vi "Destroy.vi"(8 "error in (no error)":errorcluster, 11 "reference in":refnum<class "GOOP4_Sub.lvclass">) -> (0 "error out":errorcluster, 3 "reference out":refnum<class "GOOP4_Sub.lvclass">)   [LabVIEW 2019, in "GOOP4_Sub.lvclass"]
uses:
  GOOP4_Sub.lvclass
  GOOP4_Base_class/GOOP4_Base.lvclass
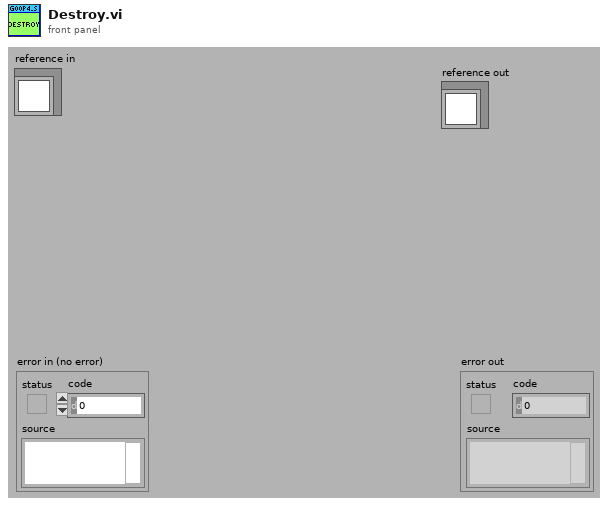
[diagram p1: front panel]
types:
  T1 = typedef "GOOP4_Sub.lvclass/ObjectAttributes.ctl" = cluster{"Str":string, "Boolean":bool}
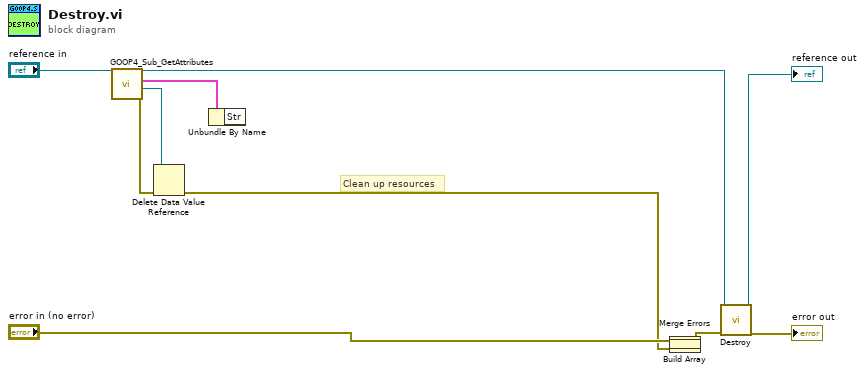
[diagram p0: block diagram]
diagram:
  # "Clean up resources"
  n1 = call "GOOP4_Sub_GetAttributes.vi"("reference in"="reference in") -> ("error out"=w8:errorcluster, "DataRef"=w4:refnum<data-value>, "Data"=w7:T1, "reference out"=w5:refnum<class "GOOP4_Sub.lvclass">)  [unwired: 7 in]
  n2 = Delete Data Value Reference(data value reference=w4, error in=w8) -> (error out=w2:errorcluster)  [unwired: 1 out]
  n3 = Unbundle By Name(w7) -> ()  [unwired: 1 out]
  n4 = Build Array("error in (no error)", w2) -> (w1:errorcluster[])
  n5 = Merge Errors(w1) -> (w11:errorcluster)
  n6 = call-parent "Destroy.vi"("error in (no error)"=w11, "reference in"=w5) -> ("error out"=→"error out":errorcluster, "reference out"=→"reference out":refnum<class "GOOP4_Sub.lvclass">)  [unwired: 8 in]
